vi "Process-Sample.vi"(8 "error in (no error)":errorcluster, 11 "Process":refnum<vi>) -> (0 "error out":errorcluster)   [LabVIEW 2016]
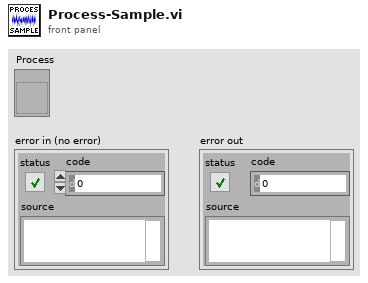
[diagram p1: front panel]
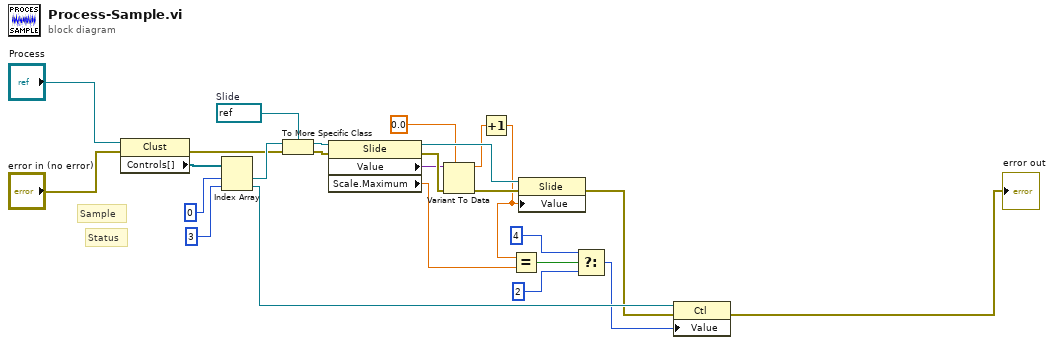
[diagram p0: block diagram]
diagram:
  w18 = refnum<vi> refnum  # Slide
  # "Status"
  # "Sample"
  n1 = property class="Clust"(reference="Process", error in="error in (no error)") -> (error out=w16:errorcluster, "Controls[]"=w14:refnum<vi>[])  [unwired: 1 out]
  n2 = Index Array(array=w14, index #1=0 ("index"), index #2=3 ("index")) -> (element #1=w17:refnum<vi>, element #2=w6:refnum<vi>)
  n3 = To More Specific Class(target class=w18, reference=w17, error in=w16) -> (specific class reference=w20:refnum<vi>, error out=w19:errorcluster)
  n4 = property class="Slide"(reference=w20, error in=w19) -> (reference out=w23:refnum<vi>, error out=w22:errorcluster, "Value"=w21:variant, "Scale.Maximum"=w12:dbl)
  n5 = Variant To Data(error in=w22, type=0.0, Variant=w21) -> (data=w11:dbl, error out=w24:errorcluster)
  n6 = Increment(x=w11) -> (x+1=w2:dbl)
  n7 = Equal?(x=w2, y=w12) -> (x = y?=w10:bool)
  n8 = property class="Slide"(reference=w23, error in=w24, "Value"=w2) -> (error out=w4:errorcluster)  [unwired: 1 out]
  n9 = Select(t=4, s=w10, f=2) -> (s? t:f=w5:i32)
  n10 = property class="Ctl"(reference=w6, error in=w4, "Value"=w5) -> (error out=→"error out":errorcluster)  [unwired: 1 out]
